vi "goal_filter.vi"(6 "Speedup":sgl, 7 "Parameters":T2={"Stimulus"={"Type"=enum."Off", "Phase"=0.0, "Amplitude"=[], "Injection point"=enum."Total pose", "Closed loop"=FALSE, "Offset"=[], "Tip -> world"=FALSE, "Frequency"=0.0, "Length"=0.0}, "Goal Filter A"={"Speedup max"=0.0, "Speedup thresh"=0.0, "Speedup nonlin"=0.0, "Filters"=[]}, "Mode controls"={"Hold"=FALSE, "Cancellation"=FALSE, "Goal filter"=FALSE, "Trigger"=FALSE}, "Manipulator type"=enum."Current piezo", "Manipulator calibration"={"Tool offsets"=[[0.0, 0.0, 36200.0]], "Handle light calibration"=[], "Base pivots"=[], "Output pivots"=[], "Length center"=0.0, "Workspace height"=[], "Workspace diameter"=[0.0, 0.0, 36200.0], "Stack travel"=400.0, "Saturation pos"=375.0, "Inverse filters"=[], "Strut length"=0.0}, "Network"={"Remote Host"="", "Send Status"=FALSE, "Send Port"=0, "Recv Commands"=FALSE, "Recv Port"=0}, "Goal Filter B"={"Speedup max"=0.0, "Speedup thresh"=0.0, "Speedup nonlin"=0.0, "Filters"=[]}, "Cancellation"={"KP"={"XY"=0.0, "Rxy"=0.0, "Z"=0.0, "Rz"=0.0}, "KI"=0.0, "KD"={"XY"=0.0, "Rxy"=0.0, "Z"=0.0, "Rz"=0.0}, "Max vel"=20.0, "Max acc"=0.001, "Int error limit"=3.0, "RCM gain"=0.0, "Bypass"=FALSE, "Degraded gain"=0.0}, "Transition time"=0.0, "Estimation"={"Link"={"Measure noise"=[], "Process noise"=[], "Alt process noise"=[], "Alt turnoff cycles"=20, "Innovation limit"=[], "Residue threshold"=0.0, "Enable"=FALSE}, "Handle"={"Measure noise"=[], "Process noise"=[], "State limits"=[], "Innovation limit"=[], "Prediction Lookahead"=0.0, "Enable"=FALSE}}} {"Transition time" format="%_3f"; "Cancellation"."Degraded gain" min=0 max=1 step=0.1 format="%#_3p"; "Cancellation"."RCM gain" min=0 max=1 step=0.1 format="%#_3p"; "Cancellation"."KD"."Rz" min=-1 max=1 step=0.01 format="%#_3p"; "Cancellation"."KD"."Rxy" min=-1 max=1 step=0.01 format="%#_3p"; "Cancellation"."KD"."Z" min=-1 max=1 step=0.01 format="%#_3p"; "Cancellation"."KD"."XY" min=-1 max=1 step=0.01 format="%#_3p"; "Cancellation"."KI" min=0 max=1 step=0.01 format="%#_3p"; "Cancellation"."KP"."Rz" min=-1 max=1 step=0.01 format="%#_3p"; "Cancellation"."KP"."Rxy" min=-1 max=1 step=0.01 format="%#_3p"; "Cancellation"."KP"."Z" min=-1 max=1 step=0.01 format="%#_3p"; "Cancellation"."KP"."XY" min=-1 max=1 step=0.01 format="%#_3p"; "Cancellation"."Max acc" format="%#_3p"; "Goal Filter B"."Filters"."V limit range" format="%_3p"; "Goal Filter B"."Filters"."V limit" format="%_3p"; "Goal Filter B"."Filters"."Upper Q" format="%_3f"; "Goal Filter B"."Filters"."Upper Fc" format="%_3p"; "Goal Filter B"."Filters"."Lower Q" format="%_3f"; "Goal Filter B"."Filters"."Scale factor" format="%_3f"; "Goal Filter B"."Filters"."Lower Fc" format="%_3p"; "Goal Filter B"."Speedup nonlin" format="%_3p"; "Goal Filter B"."Speedup thresh" format="%_3p"; "Goal Filter B"."Speedup max" format="%_3p"; "Manipulator calibration"."Strut length" format="%#_4p"; "Manipulator calibration"."Saturation pos" format="%#.1f"; "Manipulator calibration"."Stack travel" format="%#.1f"; "Manipulator calibration"."Length center" format="%#_4p"; "Manipulator calibration"."Output pivots" format="%#_6f"; "Manipulator calibration"."Base pivots" format="%#_6f"; "Manipulator calibration"."Handle light calibration" format="%#.1f"; "Goal Filter A"."Filters"."V limit range" format="%_3p"; "Goal Filter A"."Filters"."V limit" format="%_3p"; "Goal Filter A"."Filters"."Upper Q" format="%_3f"; "Goal Filter A"."Filters"."Upper Fc" format="%_3p"; "Goal Filter A"."Filters"."Lower Q" format="%_3f"; "Goal Filter A"."Filters"."Scale factor" format="%_3f"; "Goal Filter A"."Filters"."Lower Fc" format="%_3p"; "Goal Filter A"."Speedup nonlin" format="%_3p"; "Goal Filter A"."Speedup thresh" format="%_3p"; "Goal Filter A"."Speedup max" format="%_3p"; "Stimulus"."Length" min=0.0 max=100.0 step=100.0 format="%#_4p"; "Stimulus"."Frequency" min=0.0 step=100.0 format="%#_4g"; "Stimulus"."Offset" format="%#_3p"; "Stimulus"."Amplitude" format="%#_3p"; "Stimulus"."Phase" min=-180.0 max=360.0 step=100.0 format="%#.2f"}, 8 "Reset":bool, 9 "Sampling frequency":sgl=1.0 format="%0.2f", 10 "Goal position in":sgl[](array[numeric]), 11 "Goal filter":T1={"Lower Fc"=0.08, "Lower Q"=0.606, "Scale factor"=3.0, "Upper Fc"=2.0, "Upper Q"=0.606, "V limit"=1.5, "V limit range"=25.0} {"V limit range" format="%_3p"; "V limit" format="%_3p"; "Upper Q" format="%_3f"; "Upper Fc" format="%_3p"; "Lower Q" format="%_3f"; "Scale factor" format="%_3f"; "Lower Fc" format="%_3p"}) -> (1 "Goal position out":sgl[](array[numeric]))   [LabVIEW 2014]
uses:
  testing/Micron params.ctl
  testing/stimulus.ctl
  testing/injection_point.ctl
  goal_loop_parms.ctl
  testing/mode_conrols.ctl
  testing/manipulator_cal.ctl
  asap/labview/testing/probe_calibration.ctl
  host/network_params.ctl
  cancellation/sq_control_params.ctl
  cancellation/decoupled_gain.ctl
  cancellation/estimation_controls.ctl
  goal_filter_parms.ctl
panel:
  # "Locals:"
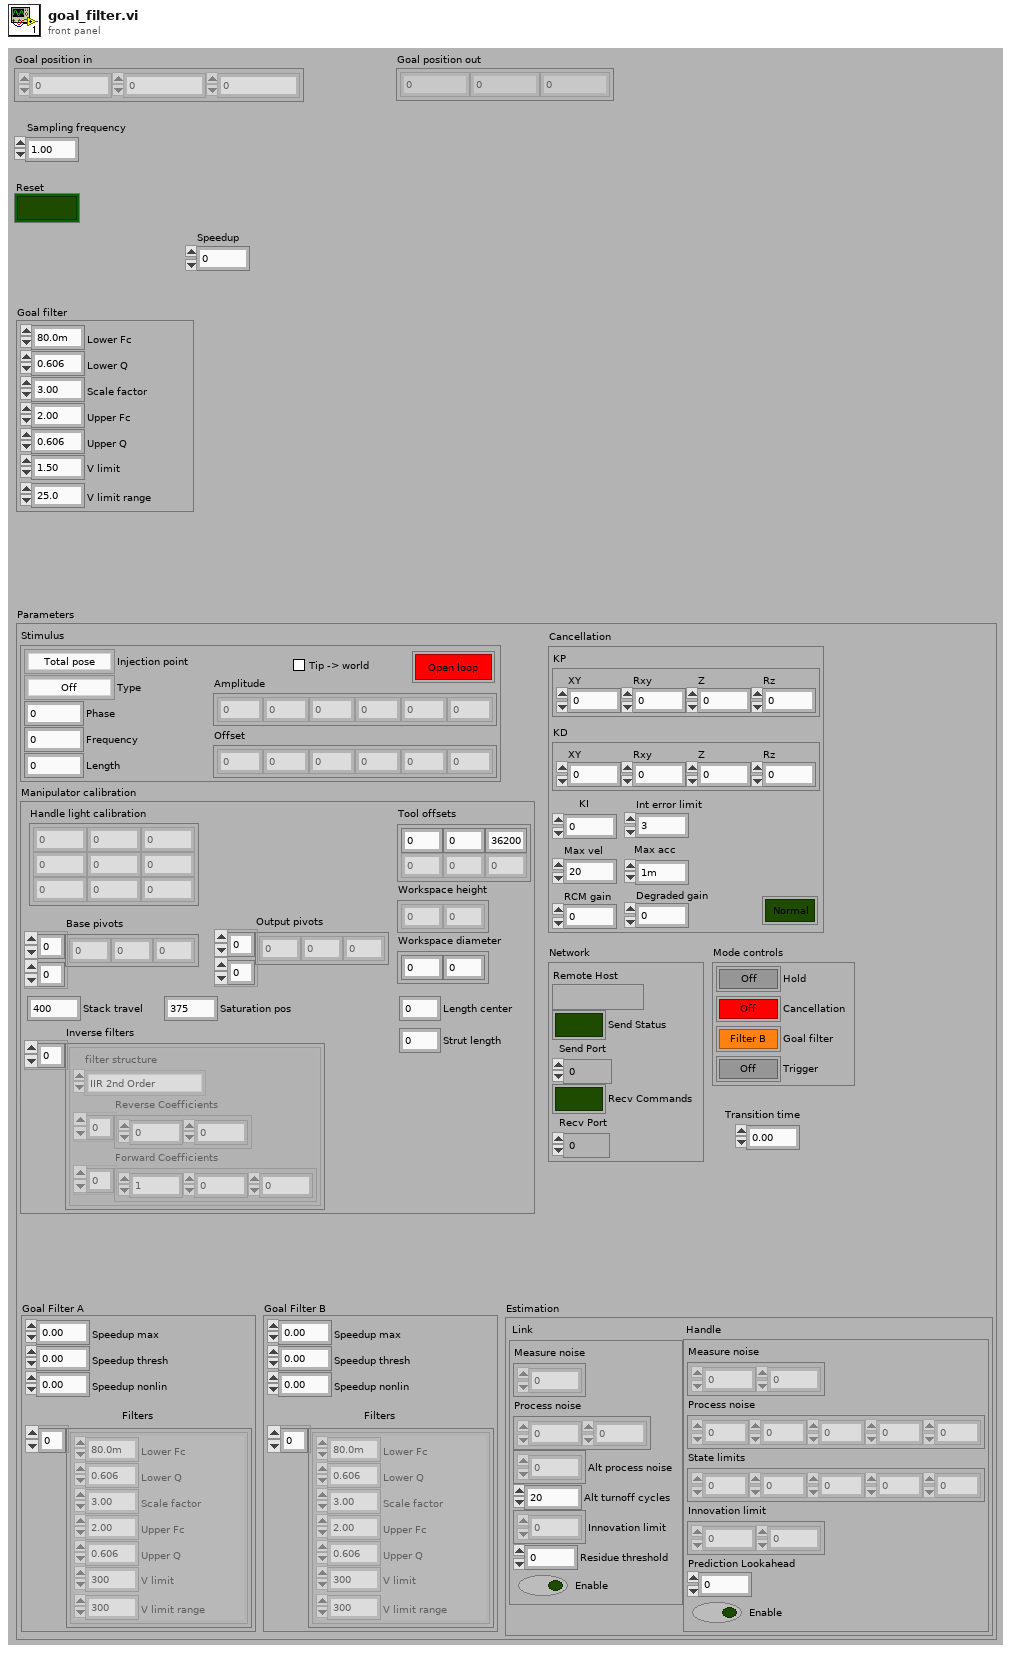
[diagram p1: front panel]
types:
  T1 = typedef "goal_filter_parms.ctl" = cluster{"Lower Fc":sgl, "Lower Q":sgl, "Scale factor":sgl, "Upper Fc":sgl, "Upper Q":sgl, "V limit":sgl, "V limit range":sgl}
  T2 = typedef "Micron params.ctl" = cluster{"Stimulus":T3, "Goal Filter A":T5, "Mode controls":T6, "Manipulator type":enum16{"Current piezo", "Voltage piezo"}, "Manipulator calibration":T7, "Network":T9, "Goal Filter B":T5, "Cancellation":T10, "Transition time":sgl, "Estimation":T12}
  T3 = typedef "stimulus.ctl" = cluster{"Type":enum16{"Off", "Step", "Sine", "Triangle", "Arbitrary"}, "Phase":dbl, "Amplitude":sgl[], "Injection point":T4, "Closed loop":bool, "Offset":sgl[], "Tip -> world":bool, "Frequency":dbl, "Length":dbl}
  T4 = typedef "injection_point.ctl" = enum16{"Total pose", "V limiter", "Goal ", "Link position", "KF link position", "Inverse kin", "Link goal", "Link error", "Controller", "Output", "Drive", "Light"}
  T5 = typedef "goal_loop_parms.ctl" = cluster{"Speedup max":sgl, "Speedup thresh":sgl, "Speedup nonlin":sgl, "Filters":cluster{"Lower Fc":sgl, "Lower Q":sgl, "Scale factor":sgl, "Upper Fc":sgl, "Upper Q":sgl, "V limit":sgl, "V limit range":sgl}[]}
  T6 = typedef "mode_conrols.ctl" = cluster{"Hold":bool, "Cancellation":bool, "Goal filter":bool, "Trigger":bool}
  T7 = typedef "manipulator_cal.ctl" = cluster{"Tool offsets":sgl[][], "Handle light calibration":T8, "Base pivots":sgl[][], "Output pivots":sgl[][], "Length center":sgl, "Workspace height":sgl[], "Workspace diameter":sgl[], "Stack travel":sgl, "Saturation pos":sgl, "Inverse filters":cluster{"filter structure":enum32{"IIR 2nd Order", "IIR 4th Order"}, "Reverse Coefficients":dbl[], "Forward Coefficients":dbl[]}[], "Strut length":sgl}
  T8 = typedef "probe_calibration.ctl" = sgl[][]
  T9 = typedef "network_params.ctl" = cluster{"Remote Host":string, "Send Status":bool, "Send Port":u16, "Recv Commands":bool, "Recv Port":u16}
  T10 = typedef "sq_control_params.ctl" = cluster{"KP":T11, "KI":sgl, "KD":T11, "Max vel":sgl, "Max acc":sgl, "Int error limit":sgl, "RCM gain":sgl, "Bypass":bool, "Degraded gain":sgl}
  T11 = typedef "decoupled_gain.ctl" = cluster{"XY":sgl, "Rxy":sgl, "Z":sgl, "Rz":sgl}
  T12 = typedef "estimation_controls.ctl" = cluster{"Link":cluster{"Measure noise":dbl[], "Process noise":dbl[], "Alt process noise":dbl[], "Alt turnoff cycles":i32, "Innovation limit":dbl[], "Residue threshold":dbl, "Enable":bool}, "Handle":cluster{"Measure noise":dbl[], "Process noise":dbl[], "State limits":dbl[], "Innovation limit":dbl[], "Prediction Lookahead":sgl, "Enable":bool}}
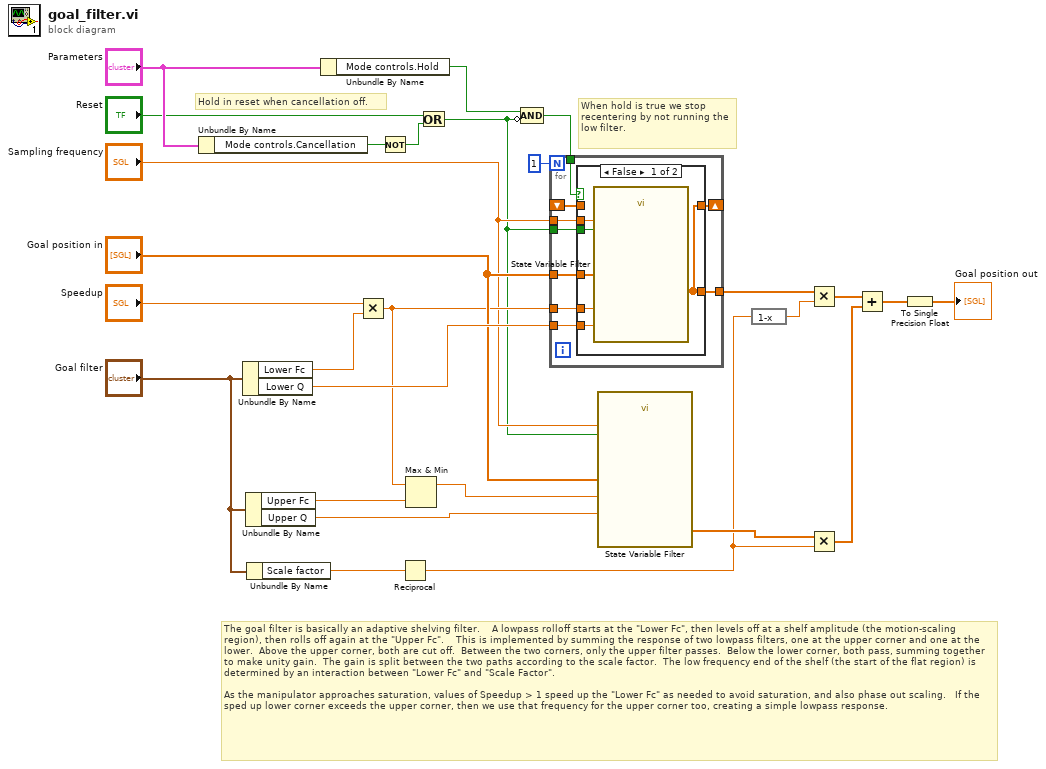
[diagram p0: block diagram]
diagram:
  # "Hold in reset when cancellation off."
  # "The goal filter is basically an adaptive shelving filter.    A lowpass rolloff starts at the \"Lower Fc\", then levels off at a shelf amplitude (the motion-scaling region), then rolls off again at the \"Upper Fc\".    This is implemented by summing the response of two lowpass filters, one at the upper corner and one at the lower.  Above the upper corner, both are cut off.  Between the two corners, only the upper filter passes.  Below the lower corner, both pass, summing together to make unity gain.  The gain is split between the two paths according to the scale factor.  The low frequency end of the shelf (the start of the flat region) is determined by an interaction between \"Lower Fc\" and \"Scale Factor\".\n\nAs the manipulator approaches saturation, values of Speedup > 1 speed up the \"Lower Fc\" as needed to avoid saturation, and also phase out scaling.   If the sped up lower corner exceeds the upper corner, then we use that frequency for the upper corner too, creating a simple lowpass response."
  # "When hold is true we stop recentering by not running the low filter."
  n1 = Unbundle By Name("Parameters") -> ("Mode controls.Cancellation"=w7:bool)
  n2 = Unbundle By Name("Goal filter") -> ("Lower Fc"=w24:sgl, "Lower Q"=w23:sgl)
  n3 = Unbundle By Name("Goal filter") -> ("Upper Fc"=w14:sgl, "Upper Q"=w12:sgl)
  n4 = Unbundle By Name("Goal filter") -> ("Scale factor"=w11:sgl)
  n5 = Unbundle By Name("Parameters") -> ("Mode controls.Hold"=w27:bool)
  n6 = Multiply(x="Speedup", y=w24) -> (x*y=w15:sgl)
  n7 = Not(x=w7) -> (.not. x?=w8:bool)
  n8 = Reciprocal(x=w11) -> (1/x=w17:sgl)
  n9 = Max & Min(x=w15, y=w14) -> (max(x,y)=w13:sgl)  [unwired: 1 out]
  n10 = Or(x="Reset", y=w8) -> (x .or. y?=w5:bool)
  n11 = Compound Arithmetic op=AND(w27, invert w5) -> (w3:bool)
  n12 = for {
    N: 1 -> [_]
    tunnel: w23 -> [w36]
    tunnel: "Goal position in" -> [w35]
    tunnel: [w34] -> w19
    tunnel: w15 -> [w33]
    tunnel: "Sampling frequency" -> [w32]
    tunnel: w5 -> [w31]
    tunnel: w3 -> [w30]
    shift-right: [w28] -> _
    shift-left: _ -> [w29]
    n13 = case shown="False" w30 {
      tunnel: w36 -> [w42 _]
      tunnel: w35 -> [w41 _]
      tunnel: [w37 w43] -> w34
      tunnel: w33 -> [w40 _]
      tunnel: w32 -> [w39 _]
      tunnel: w31 -> [w38 _]
      tunnel: w29 -> [_ w43]
      tunnel: [w37 w43] -> w28
      frame False {
        n14 = call "State Variable Filter.vi"("initialize"=w38, "Fs"=w39, "Q"=w42, "Fc"=w40, "x"=w41) -> ("Lowpass"=w37:dbl[])  [unwired: 6 out]
      }
      frame True {
      }
    }
  }
  n15 = call "State Variable Filter.vi"("initialize"=w5, "Fs"="Sampling frequency", "Q"=w12, "Fc"=w13, "x"="Goal position in") -> ("Lowpass"=w21:dbl[])  [unwired: 6 out]
  n16 = expression code="1-x"(w17) -> (w18:sgl)
  n17 = Multiply(x=w19, y=w18) -> (x*y=w16:dbl[])
  n18 = Multiply(x=w21, y=w17) -> (x*y=w20:dbl[])
  n19 = Add(x=w16, y=w20) -> (x+y=w26:dbl[])
  n20 = To Single Precision Float(number=w26) -> (single precision float=→"Goal position out":sgl[])
